vi "IDFT.vi"(1 "Input":cdb[](array[numeric])) -> (0 "Output":cdb[](array[numeric]))   [LabVIEW 2018]
uses:
  <vilib>/Analysis/baseanly.llb/Mean (CDB).vi
  <vilib>/Analysis/NI_AALBase.lvlib
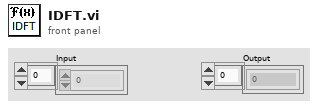
[diagram p1: front panel]
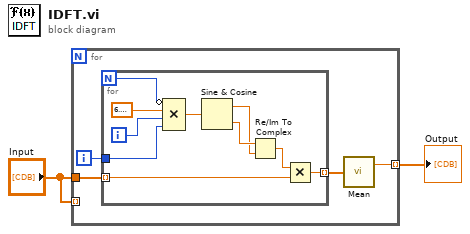
[diagram p0: block diagram]
diagram:
  n1 = for {
    tunnel: [w3] -> w2 mode=indexing
    tunnel: "Input" -> [w5]
    tunnel: "Input" -> [_] mode=indexing
    i -> [w6]
    n2 = for {
      N -> [w15]
      tunnel: [w11] -> w4 mode=indexing
      tunnel: w6 -> [w13]
      tunnel: w5 -> [w12] mode=indexing
      i -> [w14]
      n3 = Compound Arithmetic op=MULTIPLY(invert w15, 6.283185307179586, w14, w13) -> (w9:dbl)
      n4 = Sine & Cosine(0:w9) -> (1:w7:dbl, 2:w8:dbl)
      n5 = Re/Im To Complex(1:w7, 2:w8) -> (0:w10:cdb)
      n6 = Multiply(x=w10, y=w12) -> (x*y=w11:cdb)
    }
    n7 = call-poly <vilib>:"Mean.vi"("X"=w4) -> ("mean"=w3:cdb)  [unwired: 1 out]
  }
  "Output" <- w2
